vi "Run Hologram Engine.vi"() -> (0 "status":bool)   [LabVIEW 2020]
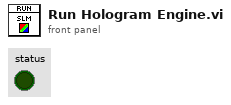
[diagram p1: front panel]
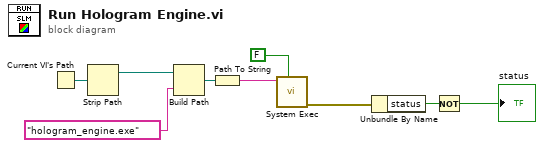
[diagram p0: block diagram]
diagram:
  n1 = Current VI's Path() -> (path=w5:path)
  n2 = Strip Path(path=w5) -> (stripped path=w6:path)  [unwired: 1 out]
  n3 = Build Path(base path=w6, name or relative path="hologram_engine.exe") -> (appended path=w9:path)
  n4 = Path To String(path=w9) -> (string=w8:string)
  n5 = call <vilib>:"System Exec.vi"("wait until completion? (T)"=FALSE, "command line"=w8) -> ("error out"=w3:errorcluster)  [unwired: 6 in, 3 out]
  n6 = Unbundle By Name(w3) -> ("status"=w2:bool)
  n7 = Not(x=w2) -> (.not. x?=→"status":bool)
